vi "Block Write Multiple Iterator.vi"(8 "error in (no error)":errorcluster, 9 "Iterations (1000)":i32=1000, 10 "Channel Counts":i32[](array[numeric]), 11 "GE 5565PIORC in":refnum<class "GE 5565PIORC.lvclass">) -> (0 "error out":errorcluster, 1 "Histograms":T1(array[cluster]), 2 "Metrics":T2[](array[typedef]) {"Transfer Rate" format="%.2pB/s"; "Duration Std. Dev." format="%.0f µs"; "Duration Average" format="%.0f µs"}, 3 "GE 5565PIORC out":refnum<class "GE 5565PIORC.lvclass">)   [LabVIEW 2016]
uses:
  Source/GE 5565PIORC/GE 5565PIORC.lvclass
  Controls/Throughput Metrics.ctl
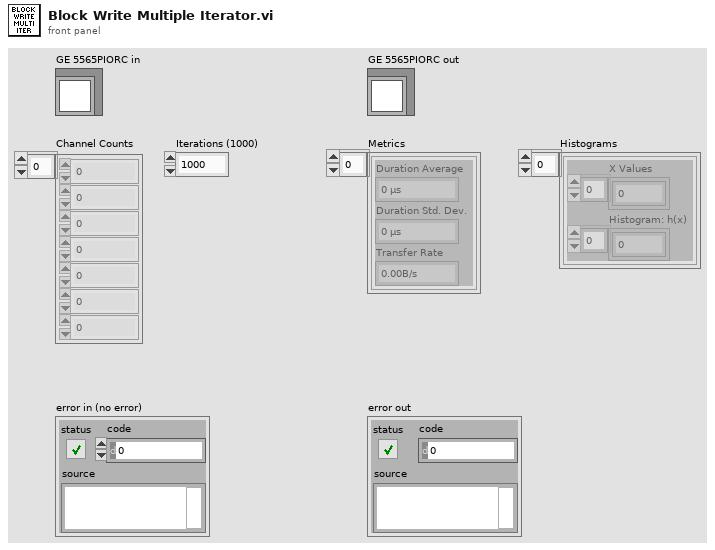
[diagram p1: front panel]
types:
  T1 = cluster{"X Values":dbl[], "Histogram: h(x)":i32[]}[]
  T2 = typedef "Throughput Metrics.ctl" = cluster{"Duration Average":u32, "Duration Std. Dev.":u32, "Transfer Rate":dbl}
  T3 = cluster{"X Values":dbl[], "Histogram: h(x)":i32[]}
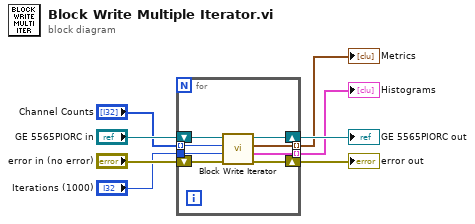
[diagram p0: block diagram]
diagram:
  n1 = for {
    shift-right: [w13] -> w5
    shift-left: "GE 5565PIORC in" -> [w16]
    shift-right: [w14] -> w6
    shift-left: "error in (no error)" -> [w15]
    tunnel: "Channel Counts" -> [w9] mode=indexing
    tunnel: "Iterations (1000)" -> [w12]
    tunnel: [w11] -> w2 mode=indexing
    tunnel: [w10] -> w1 mode=indexing
    n2 = call "Block Write Iterator.vi"("error in (no error)"=w15, "Iterations (1000)"=w12, "Channel Count"=w9, "GE 5565PIORC in"=w16) -> ("error out"=w14:errorcluster, "Histogram Graph"=w10:T3, "Metrics"=w11:T2, "GE 5565PIORC out"=w13:refnum<class "GE 5565PIORC.lvclass">)  [unwired: 4 in]
  }
  "error out" <- w6
  "GE 5565PIORC out" <- w5
  "Metrics" <- w2
  "Histograms" <- w1
